vi "WriteASCIIFile.vi"(5 "T":T1={"Error"={"status"=FALSE, "code"=0, "source"=""}, "Test Info"={"Test Name"="", "Tester"=""}, "test data"=[{"t0"=timestamp(0 s since 1904-01-01), "dt"=1.0, "Y"=[]}, {"t0"=timestamp(0 s since 1904-01-01), "dt"=1.0, "Y"=[]}, {"t0"=timestamp(0 s since 1904-01-01), "dt"=1.0, "Y"=[]}, {"t0"=timestamp(0 s since 1904-01-01), "dt"=0.001, "Y"=[]}], "Index Vibration Waveform"={"t0"=timestamp(0 s since 1904-01-01), "dt"=1.0, "Y"=[]}, "report information"={"Test Info"={"Test Name"="", "Tester"=""}, "temp chart 2"=refnum, "P chart 2"=refnum}, "TdmsInfo"={"Read Chan Name"="", "Vibr Chn Name"=[], "Read Group Name"="", "Vibr Group Name"=[]}}, 7 "file (use dialog)":path, 8 "error in (no error)":errorcluster, 9 "data":waveform(dbl)[](array[waveform]), 10 "格式":string, 11 "chanel name":string[](array[string])) -> (0 "error out":errorcluster)   [LabVIEW 2011]
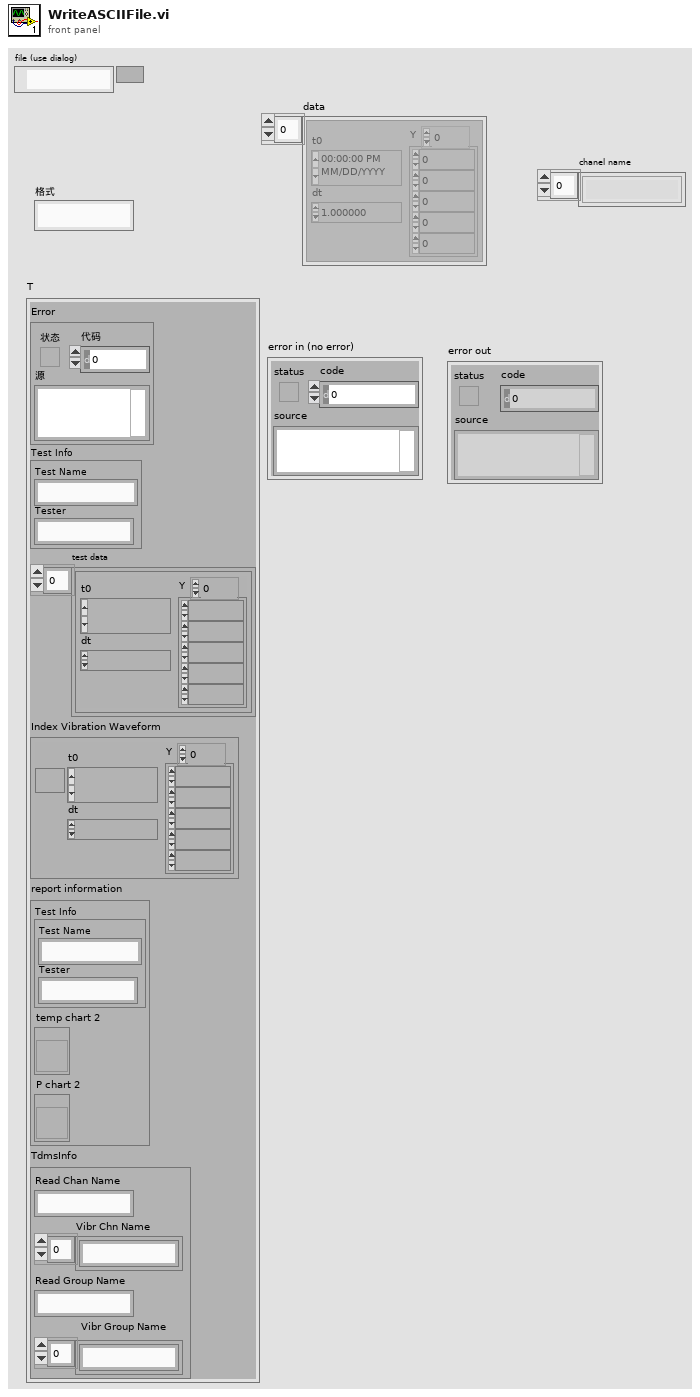
[diagram p1: front panel]
types:
  T1 = typedef "数据回放蔟0.ctl" = cluster{"Error":errorcluster, "Test Info":cluster{"Test Name":string, "Tester":string}, "test data":waveform(dbl)[], "Index Vibration Waveform":waveform(dbl), "report information":cluster{"Test Info":cluster{"Test Name":string, "Tester":string}, "temp chart 2":refnum<vi>, "P chart 2":refnum<vi>}, "TdmsInfo":cluster{"Read Chan Name":string, "Vibr Chn Name":string[], "Read Group Name":string, "Vibr Group Name":string[]}}
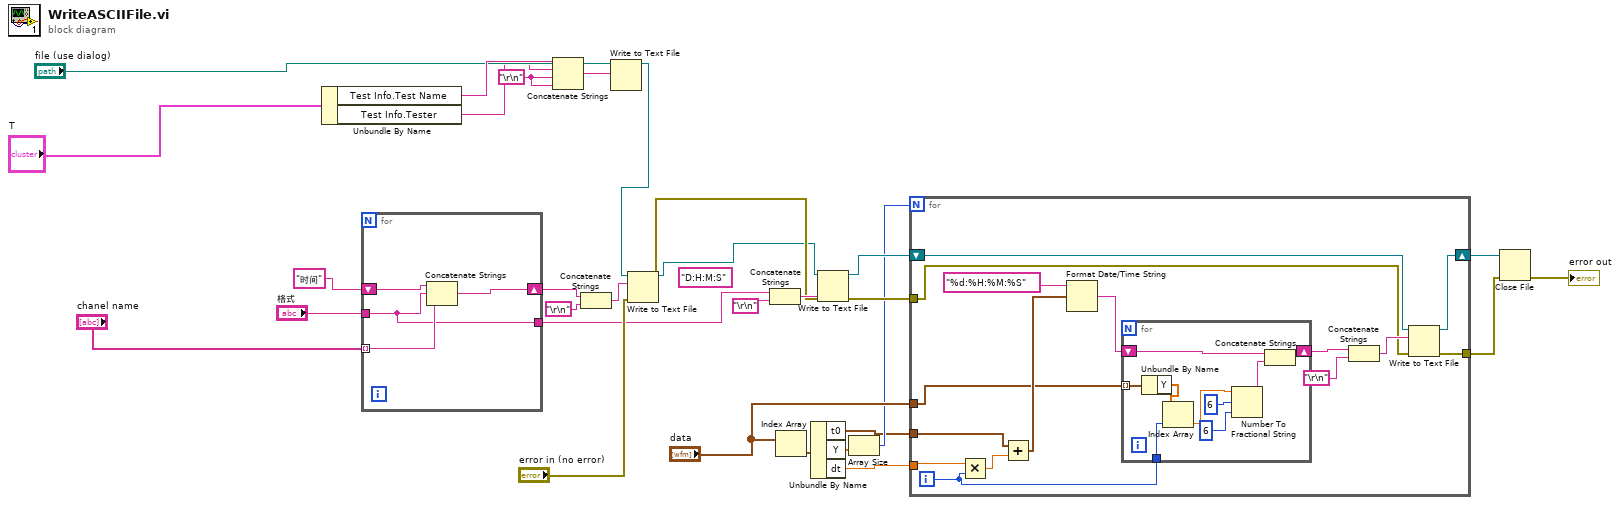
[diagram p0: block diagram]
diagram:
  w7 = "\r\n"
  (unwired) "D:H:M:S"
  n1 = Unbundle By Name("T") -> ("Test Info.Test Name"=w10:string, "Test Info.Tester"=w1:string)
  n2 = for {
    tunnel: "chanel name" -> [w32] mode=indexing
    shift-right: [w33] -> w27
    shift-left: "时间" -> [w34]
    tunnel: "格式" -> [w31]
    tunnel: [w31] -> w6
    n3 = Concatenate Strings(w34, w31, w32) -> (w33:string)
  }
  n4 = Concatenate Strings(w10, w1, w7, w7) -> (w8:string)
  n5 = Concatenate Strings(w27, "\r\n") -> (w28:string)
  n6 = Write to Text File(file (use dialog)="file (use dialog)", text=w8) -> (refnum out=w4:refnum<file>)  [unwired: 1 in, 3 out]
  n7 = Write to Text File(file (use dialog)=w4, text=w28, error in="error in (no error)") -> (refnum out=w5:refnum<file>, error out=w19:errorcluster)  [unwired: 2 out]
  n8 = Concatenate Strings(w6, "\r\n") -> (w24:string)
  n9 = Index Array(array="data") -> (element=w15:waveform(dbl))  [unwired: 1 in]
  n10 = Unbundle By Name(w15) -> ("t0"=w11:timestamp, "Y"=w14:dbl[], "dt"=w12:dbl)
  n11 = Write to Text File(file (use dialog)=w5, text=w24, error in=w19) -> (refnum out=w23:refnum<file>, error out=w20:errorcluster)  [unwired: 2 out]
  n12 = Array Size(array=w14) -> (size(s)=w13:i32)
  n13 = for {
    N: w13 -> [_]
    shift-right: [w45] -> w22
    shift-left: w23 -> [w46]
    tunnel: [w42] -> w21
    tunnel: w20 -> [w41]
    tunnel: "data" -> [w36]
    tunnel: w12 -> [w40]
    tunnel: w11 -> [w38]
    i -> [w35]
    n14 = Multiply(x=w40, y=w35) -> (x*y=w39:dbl)
    n15 = Add(x=w38, y=w39) -> (x+y=w37:timestamp)
    n16 = Format Date/Time String(time format string (%c)="%d:%H:%M:%S", seconds (now)=w37) -> (date/time string=w44:string)  [unwired: 1 out]
    n17 = for {
      shift-right: [w54] -> w49
      shift-left: w44 -> [w58]
      tunnel: w36 -> [w53] mode=indexing
      tunnel: w35 -> [w51]
      n18 = Unbundle By Name(w53) -> ("Y"=w52:dbl[])
      n19 = Index Array(array=w52, index=w51) -> (element=w50:dbl)
      n20 = Number To Fractional String(number=w50, width (-)=i16 6, precision (6)=i16 6) -> (F-format string=w55:string)  [unwired: 1 out]
      n21 = Concatenate Strings(w58, w55) -> (w54:string)
    }
    n22 = Concatenate Strings(w49, "\r\n") -> (w47:string)
    n23 = Write to Text File(file (use dialog)=w46, text=w47, error in=w41) -> (refnum out=w45:refnum<file>, error out=w42:errorcluster)  [unwired: 2 out]
  }
  n24 = Close File(refnum=w22, error in=w21) -> (error out=→"error out":errorcluster)  [unwired: 1 out]
